vi "MAN_Report.vi"(8 "error in (no error)":errorcluster, 11 "Ref In":T1={"MS SQL Connection"=refnum, "UDL File"=path "", "Time"="", "DCODE"="", "WIP+1"=0, "MC No?"=0, "POKAYOKE?"=FALSE, "Expected Result"="", "Result [Status]"="", "Clock"=0.0, "RFID"="", "WIP Queue"=refnum, "TS Parameter"={"ProfitCenterCode"="", "LineCode"="", "WorkOrderNumber"="", "Model"="", "Model_with_Prefix"="", "VendorCode"="", "SetParameterDateCode"="", "PokaYoke"=0, "Target"=1, "Live_DateCode"="", "CustomerPartNumber"="", "Hand"="", "sBarcode"=FALSE, "FCA"=0, "Ent_Stamp"=timestamp(0 s since 1904-01-01), "STS_CD"=0.0}, "Data_Queue"=[], "RFID Serial No."=""} {"TS Parameter"."FCA" format="%01d"; "TS Parameter"."Target" min=1 max=100000; "TS Parameter"."PokaYoke" min=0 max=1}) -> (0 "error out":errorcluster)   [LabVIEW 2020]
uses:
  Controls/TD SQL.ctl
  <vilib>/addons/database/Connection.llb/Conn ObjectReference.ctl
  Controls/WIP_State.ctl
  Controls/TS_Parameter.ctl
  <vilib>/addons/database/_DB Variant To Data/Database Variant To Data.xnode
  <vilib>/addons/database/NI_Database_API.lvlib
panel:
  in  "Exit":bool
  in  "Report":i32(listbox)
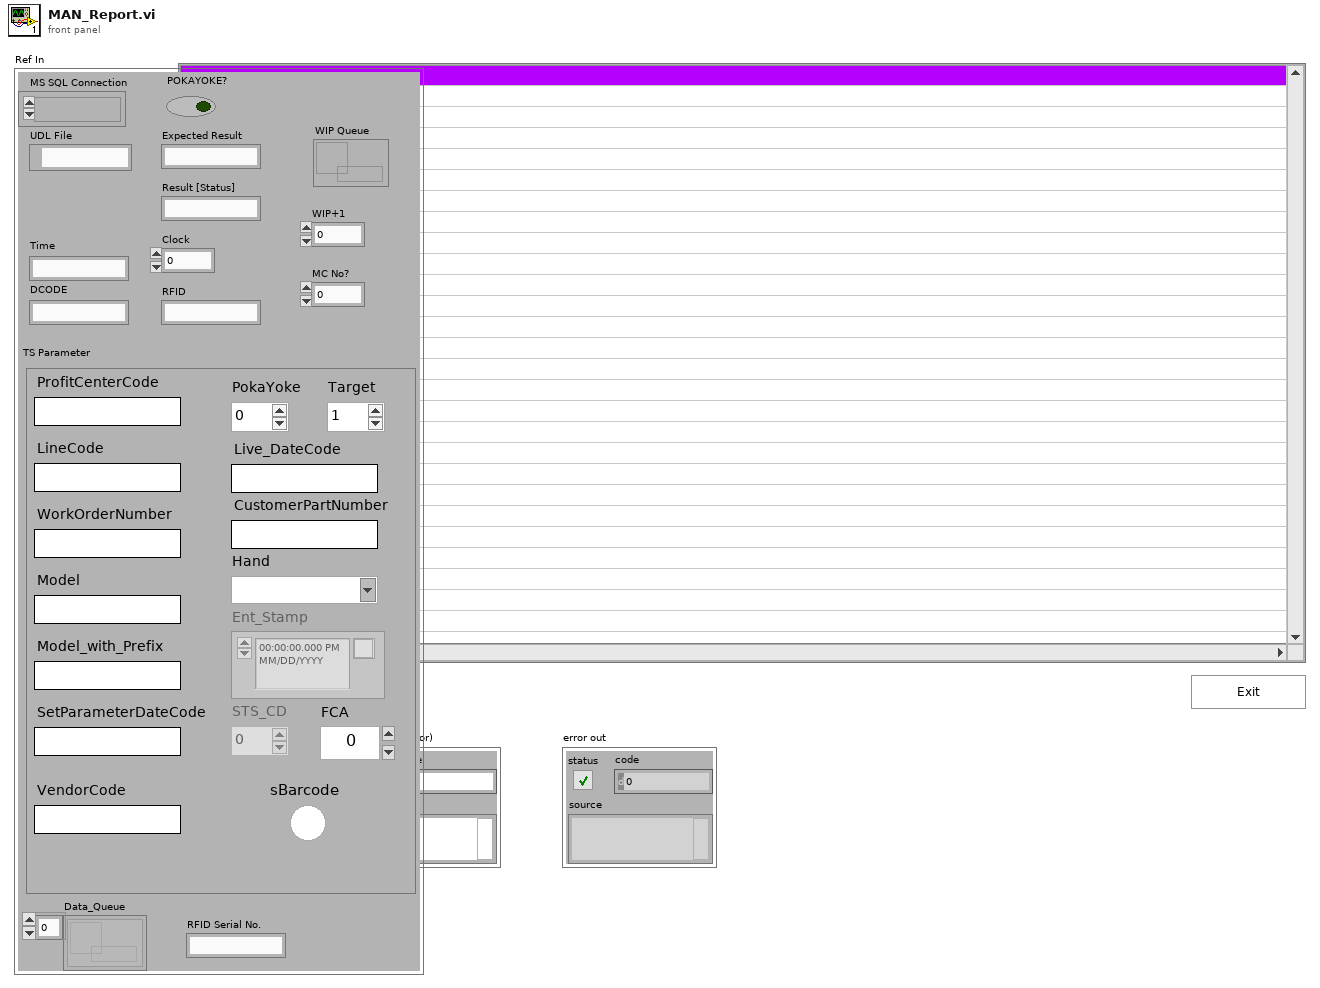
[diagram p1: front panel]
types:
  T1 = typedef "TD SQL.ctl" = cluster{"MS SQL Connection":T2, "UDL File":path, "Time":string, "DCODE":string, "WIP+1":i64, "MC No?":i32, "POKAYOKE?":bool, "Expected Result":string, "Result [Status]":string, "Clock":dbl, "RFID":string, "WIP Queue":refnum<queue>, "TS Parameter":T3, "Data_Queue":refnum<queue>[], "RFID Serial No.":string}
  T2 = typedef "NI_Database_API.lvlib/Conn ObjectReference.ctl" = refnum<k1>
  T3 = typedef "TS_Parameter.ctl" = cluster{"ProfitCenterCode":string, "LineCode":string, "WorkOrderNumber":string, "Model":string, "Model_with_Prefix":string, "VendorCode":string, "SetParameterDateCode":string, "PokaYoke":i32, "Target":i32, "Live_DateCode":string, "CustomerPartNumber":string, "Hand":string, "sBarcode":bool, "FCA":i32, "Ent_Stamp":timestamp, "STS_CD":dbl}
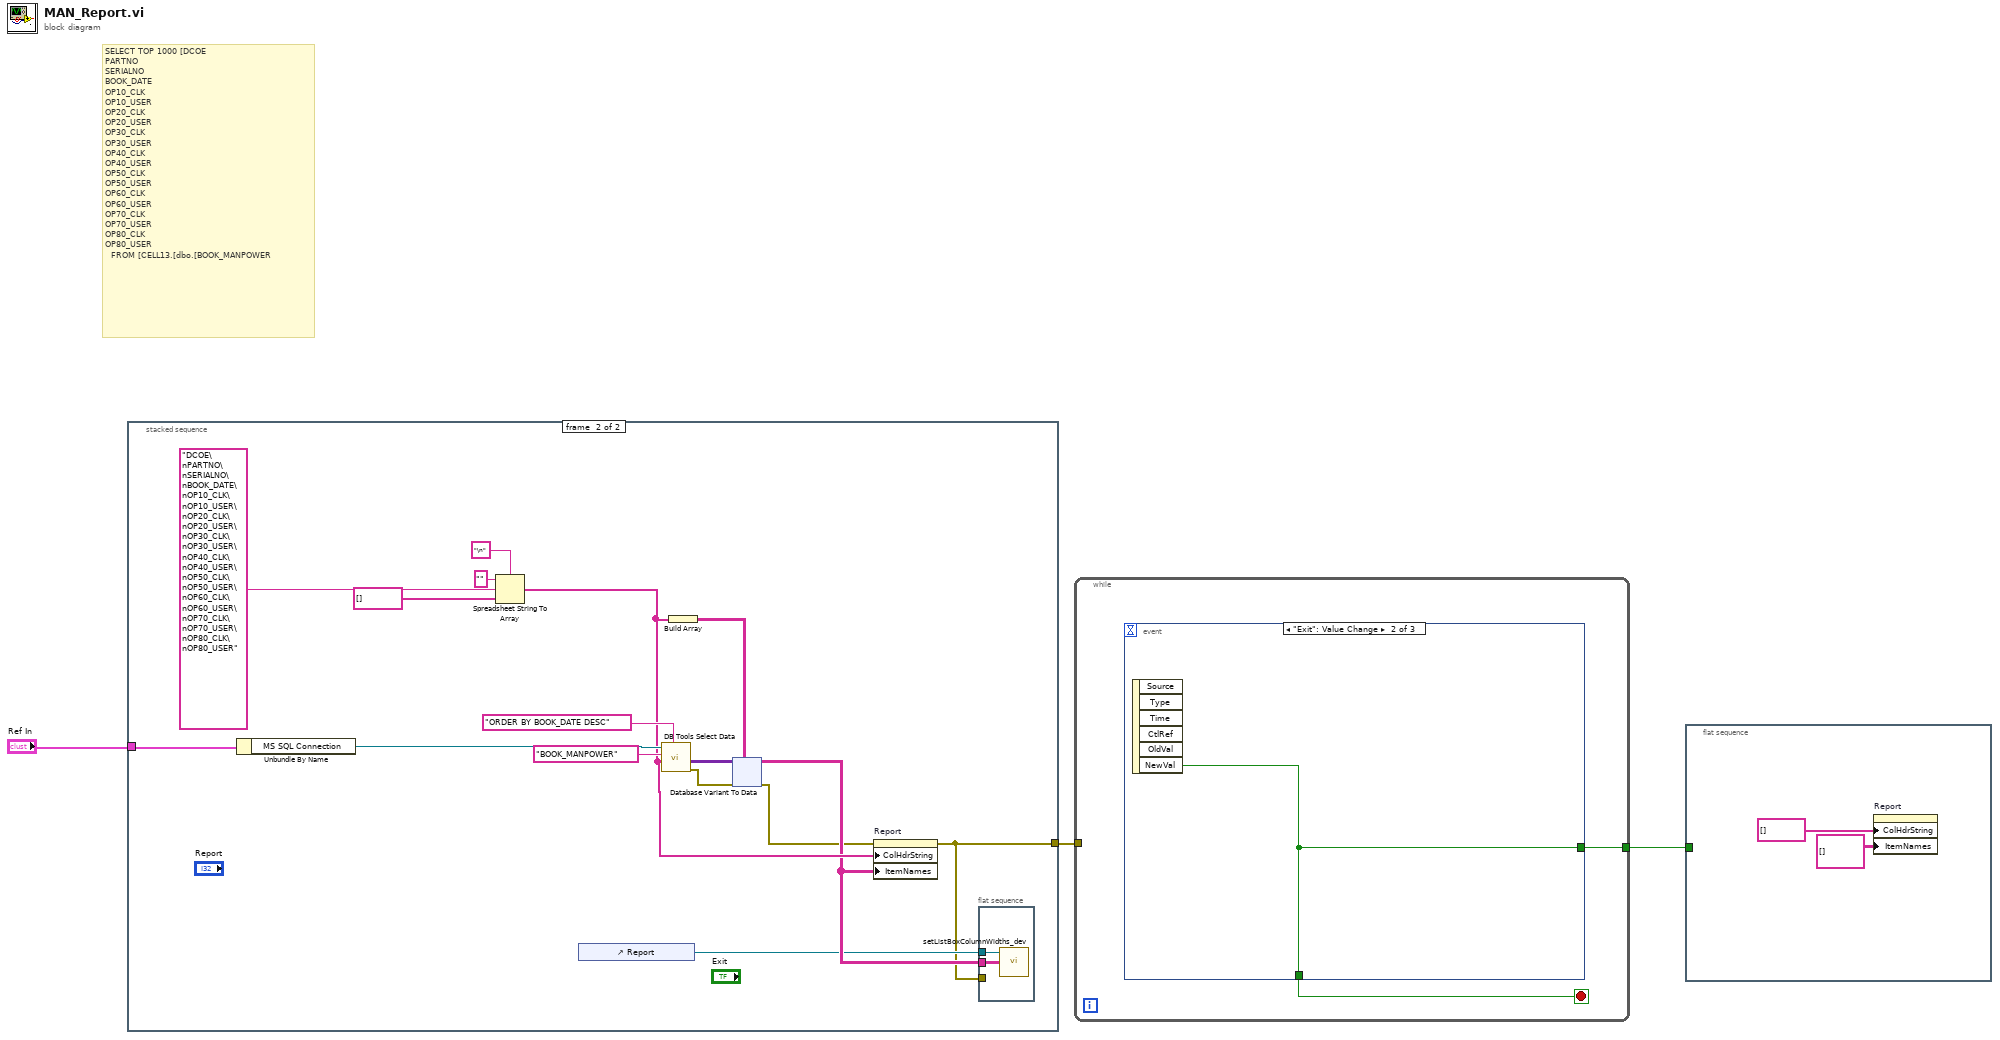
[diagram p0: block diagram]
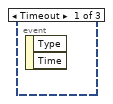
[diagram p2: hidden frame]
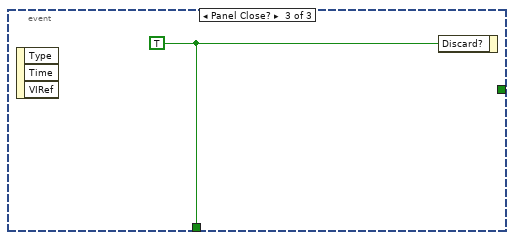
[diagram p3: hidden frame]
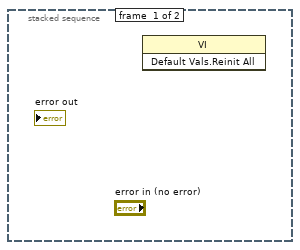
[diagram p4: hidden frame]
diagram:
  # "SELECT TOP 1000 [DCOE\nPARTNO\nSERIALNO\nBOOK_DATE\nOP10_CLK\nOP10_USER\nOP20_CLK\nOP20_USER\nOP30_CLK\nOP30_USER\nOP40_CLK\nOP40_USER\nOP50_CLK\nOP50_USER\nOP60_CLK\nOP60_USER\nOP70_CLK\nOP70_USER\nOP80_CLK\nOP80_USER\n  FROM [CELL13.[dbo.[BOOK_MANPOWER"
  n1 = stacked-sequence {
    tunnel: "Ref In" -> [_ w4]
    tunnel: [_ w5] -> w3
    frame #0 {
      n2 = invoke class="VI" method="Default Vals.Reinit All"() -> ()  [unwired: 3 in, 3 out]
    }
    frame #1 {
      n3 = Unbundle By Name(w4) -> ("MS SQL Connection"=w19:T2)
      n4 = Spreadsheet String To Array(delimiter (Tab)="\n", format string="", spreadsheet string="DCOE\nPARTNO\nSERIALNO\nBOOK_DATE\nOP10_CLK\nOP10_USER\nOP20_CLK\nOP20_USER\nOP30_CLK\nOP30_USER\nOP40_CLK\nOP40_USER\nOP50_CLK\nOP50_USER\nOP60_CLK\nOP60_USER\nOP70_CLK\nOP70_USER\nOP80_CLK\nOP80_USER", array type (2D Dbl)=string[] []) -> (array=w10:string[])
      n5 = control-ref of="Report"() -> (w8:refnum<vi>)
      n6 = call <vilib>:"DB Tools Select Data.vi"("condition"="ORDER BY BOOK_DATE DESC", "columns"=w10, "table"="BOOK_MANPOWER", "connection reference"=w19) -> ("error out"=w7:errorcluster, "data"=w13:variant[][])  [unwired: 2 in, 1 out]
      n7 = Build Array(w10) -> (w12:string[][])
      n8 = xnode "Database Variant To Data"("database variant"=w13, "error in (no error)"=w7, "type"=w12) -> ("data"=w9:string[][], "error out"=w6:errorcluster)
      n9 = property on="Report" class="MCListbox (strict)"(error in=w6, "ColHdrString"=w10, "ItemNames"=w9) -> (error out=w5:errorcluster)  [unwired: 1 in, 1 out]
      n10 = flat-sequence {
        tunnel: w9 -> [w21]
        tunnel: w8 -> [w20]
        tunnel: w5 -> [_]
        frame #0 {
          n11 = call "setListBoxColumnWidths_dev.vi"("table data"=w21, "MCListbox Refnum"=w20) -> ()  [unwired: 1 in]
        }
      }
    }
  }
  n12 = while {
    tunnel: w3 -> [_]
    tunnel: [w66] -> w1
    stop <- w67 stop-if-true
    n13 = event shown="[1] \"Exit\": Value Change" {
      selector: _ -> [_ _ _]
      dyn-events: _ -> [_ _ _]
      timeout: _ -> [_ _ _]
      tunnel: [_ w68 w69] -> w67
      tunnel: [_ w68 _] -> w66
      event Timeout {
        n14 = event-data() -> ()  [unwired: 1 in, 2 out]
      }
      event "Exit": Value Change {
        n15 = event-data() -> ("NewVal"=w68:bool)  [unwired: 1 in, 5 out]
      }
      event Panel Close? {
        w69 = TRUE ("Discard?")
        n16 = event-data() -> ()  [unwired: 1 in, 3 out]
        n17 = event-data("Discard?"=w69) -> ()  [unwired: 1 in, 1 out]
      }
    }
  }
  n18 = flat-sequence {
    tunnel: w1 -> [_]
    frame #0 {
      n19 = property on="Report" class="MCListbox (strict)"("ColHdrString"=string[] [] ("Column Header Strings[]"), "ItemNames"=string[][] [] ("Item Names")) -> ()  [unwired: 2 in, 2 out]
    }
  }
